vi "HWdespike_Pre_Analysis_Plugin.vi"() -> ()   [LabVIEW 2021]
uses:
  <vilib>/Analysis/baseanly.llb/Mean (DBL).vi
  Globals/Meas_global.vi
  <vilib>/Analysis/NI_AALBase.lvlib
panel:
  in  "minVelocity":dbl=1.5 format="%#_13g"
  in  "maxVelocity":dbl=22.0 format="%#_13g"
  # "Clamps Hotwire velocities outside specified range to be mean of entire signal"
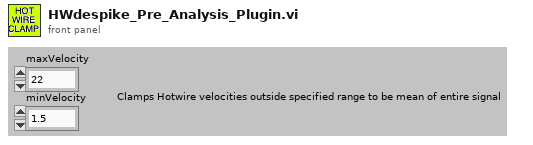
[diagram p1: front panel]
types:
  T1 = typedef "Analysis_info_cluster.ctl" = cluster{"Colour":u32, "Inst type":T2, "Inst name":string, "Symbol":string, "Code name":string, "Extra Info":string, "Inst Array":T3, "Extra Titles":string[], "Extra Values":string[], "U":dbl, "u^2":dbl, "u^3":dbl, "u^4":dbl, "Skew_u":dbl, "Kurt_u":dbl, "Sd Error in Mean":dbl, "% u'/U":dbl, "X":dbl, "Y":dbl, "Z":dbl, "Timescale integral Estimate":dbl, "Sd Error in Variance":dbl, "Calib File":path, "Calib Constants":dbl[], "Output Position":bool, "Stats":enum16{"None", "Basic", "Full"}, "Av Sampling Rate":dbl, "Av No of Samples":dbl, "Total Meas Time (s)":dbl, "ADAM Ch Name":string, "Max value":dbl, "Min value":dbl, "Req Sample Rate Hz":dbl, "Sync Delay Time (s)":dbl, "Ch No":i16, "Device":string, "Use Latest Calib":bool, "Port":string, "Metadata Ch Names":string[], "Metadata Ch Values":string[], "Label":string}
  T2 = typedef "Inst_type.ctl" = enum16{"Raw voltage", "Raw with zero offsetting", "Propeller anemometer", "Pressure Transducer", "Pitot-static tube", "Hot wire", "Cross wire 1", "Cross wire 2", "Generic Linear", "Generic Polynomial", "Generic BackPoly", "Fast FID", "Thermocouple", "Cold wire", "Pulsed Wire", "LDA Vel", "LDA Tran time", "LDA Arr time", "Microphone"}
  T3 = typedef "Instrument_Array.ctl" = enum16{"PWA", "LDA", "Analogue"}
  T4 = typedef "Time_Trace_Cluster.ctl" = cluster{"Weighting":dbl[], "Voltage":dbl[], "Eng Values":dbl[]}
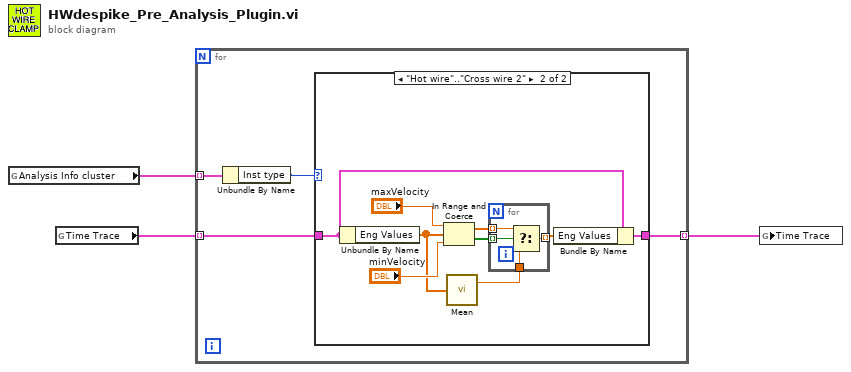
[diagram p0: block diagram]
diagram:
  n1 = global read "Meas_global.vi" "Analysis Info cluster"() -> (w3:T1[])
  n2 = global read "Meas_global.vi" "Time Trace"() -> (w2:T4[])
  n3 = for {
    tunnel: w3 -> [w7] mode=indexing
    tunnel: w2 -> [w5] mode=indexing
    tunnel: [w4] -> w1 mode=indexing
    n4 = Unbundle By Name(w7) -> ("Inst type"=w6:T2)
    n5 = case shown="\"Hot wire\"..\"Cross wire 2\"" w6 {
      tunnel: w5 -> [w8 w10]
      tunnel: [w8 w11] -> w4
      frame "Raw voltage", Default {
      }
      frame "Hot wire".."Cross wire 2" {
        n6 = Unbundle By Name(w10) -> ("Eng Values"=w12:dbl[])
        n7 = In Range and Coerce(upper limit="maxVelocity", x=w12, lower limit="minVelocity") -> (coerced(x)=w15:dbl[], In Range?=w17:bool[])
        n8 = call-poly <vilib>:"Mean.vi"("X"=w12) -> ("mean"=w16:dbl)  [unwired: 1 out]
        n9 = for {
          tunnel: w15 -> [w21] mode=indexing
          tunnel: w16 -> [w20]
          tunnel: w17 -> [w19] mode=indexing
          tunnel: [w18] -> w9 mode=indexing
          n10 = Select(t=w21, s=w19, f=w20) -> (s? t:f=w18:dbl)
        }
        n11 = Bundle By Name(cluster=w10, "Eng Values"=w9) -> (w11:T4)
      }
    }
  }
  n12 = global write "Meas_global.vi" "Time Trace"(w1) -> ()
